vi "WPI_DriverStationStop VI Asynchronous.vi"(11 "VI Refnum":refnum<vi>) -> (0 "error out":errorcluster)   [LabVIEW 2017]
doc: "This software is licensed. Open the labview\\readme\\WPI Robotics Library Open Source License.txt file for more information."
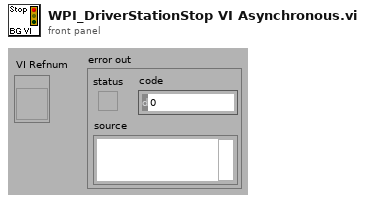
[diagram p1: front panel]
types:
  T1 = enum16{"Add", "Remove", "Acquire All", "Release All"}
  T2 = enum32{"Bad", "Idle", "Run top level", "Running"}
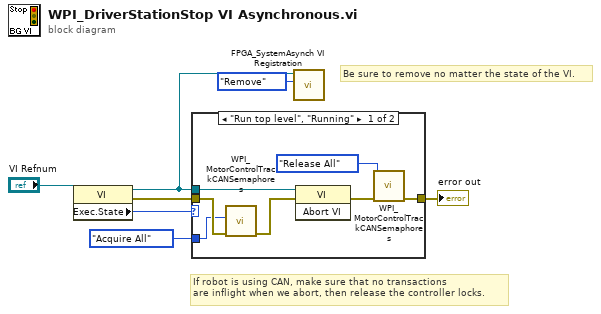
[diagram p0: block diagram]
diagram:
  # "If robot is using CAN, make sure that no transactions\nare inflight when we abort, then release the controller locks."
  # "Be sure to remove no matter the state of the VI."
  n1 = property class="VI"(reference="VI Refnum") -> (reference out=w2:refnum<vi>, error out=w5:errorcluster, "Exec.State"=w6:T2)  [unwired: 1 in]
  n2 = case shown="\"Run top level\", \"Running\"" w6 {
    tunnel: w2 -> [w14 _]
    tunnel: w5 -> [w12 w15]
    tunnel: [w10 w15] -> w4
    tunnel: T1."Acquire All" ("Operation") -> [w8 _]
    frame "Run top level", "Running" {
      n3 = call <vilib>:"WPI_MotorControlTrackCANSemaphores.vi"("error in (no error)"=w12, "Operation"=w8) -> ("error out"=w11:errorcluster)  [unwired: 9 in]
      n4 = invoke class="VI" method="Abort VI"(reference=w14, error in=w11) -> (error out=w13:errorcluster)  [unwired: 1 in, 2 out]
      n5 = call <vilib>:"WPI_MotorControlTrackCANSemaphores.vi"("error in (no error)"=w13, "Operation"=T1."Release All") -> ("error out"=w10:errorcluster)  [unwired: 9 in]
    }
    frame "Bad", "Idle" {
    }
  }
  "error out" <- w4
  n6 = call <vilib>:"FPGA_SystemAsynch VI Registration.vi"("Operation"=enum16{"Get", "Add", "Remove"}."Remove", "VI Refnum"=w2) -> ()  [unwired: 10 out]
